vi "Generate Filter Rule XML.vi"(11 "Filter Rules":T1[](array[typedef])) -> (3 "Filter Rule XML":string)   [LabVIEW 2015, in "NI_AWS_S3.lvlib"]
uses:
  NI_AWS_S3.lvlib
  Core/HTTP Request/Name Value Pair.ctl
  Core/HTTP Request/HTTP Request.lvclass
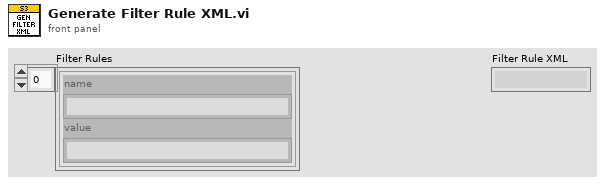
[diagram p1: front panel]
types:
  T1 = typedef "NI_AWS_Core.lvlib/HTTP Request.lvclass/Name Value Pair.ctl" = cluster{"name":string, "value":string}
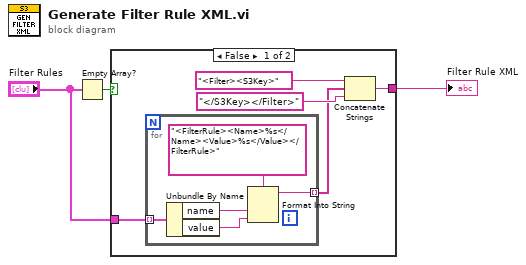
[diagram p0: block diagram]
diagram:
  n1 = Empty Array?(array="Filter Rules") -> (empty?=w1:bool)
  n2 = case shown="False" w1 {
    tunnel: "Filter Rules" -> [w5 _]
    tunnel: [w6 _] -> w3
    frame False {
      n3 = for {
        tunnel: w5 -> [w13] mode=indexing
        tunnel: [w9] -> w4 mode=indexing
        n4 = Unbundle By Name(w13) -> ("name"=w12:string, "value"=w11:string)
        n5 = Format Into String(format string="<FilterRule><Name>%s</Name><Value>%s</Value></FilterRule>", w12, w11) -> (resulting string=w9:string)  [unwired: 2 in, 1 out]
      }
      n6 = Concatenate Strings("<Filter><S3Key>", w4, "</S3Key></Filter>") -> (w6:string)
    }
    frame True {
    }
  }
  "Filter Rule XML" <- w3
